vi "Queues fgv.vi"(7 "Modes":T1, 8 "error in (no error)":errorcluster) -> (0 "error in (no error) 2":errorcluster, 1 "DAQ":refnum<queue>, 2 "Camera":refnum<queue>, 3 "Ivium":refnum<queue>)   [LabVIEW 2016]
uses:
  Controls/Queue modes.ctl
  Controls/State control cluster.ctl
  Controls/States.ctl
  Webcam/Controls/Camera queue.ctl
  Webcam/Controls/Camera states.ctl
  DAQ/Controls/DAQ queue.ctl
  DAQ/Controls/Queue states.ctl
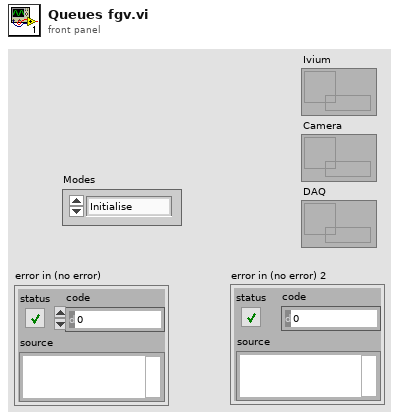
[diagram p1: front panel]
types:
  T1 = typedef "Queue modes.ctl" = enum16{"Initialise", "Destroy", "Get"}
  T2 = typedef "DAQ queue.ctl" = cluster{"Sate":T3, "Data":variant}
  T3 = typedef "Queue states.ctl" = enum16{"Shutdown", "Save data", "Record", "Read", "Setup", "Zero", "Connect", "Initialise"}
  T4 = typedef "Camera queue.ctl" = cluster{"State":T5, "Data":variant}
  T5 = typedef "Camera states.ctl" = enum16{"Initialise", "Setup", "Connect", "Snap", "Close", "Shutdown"}
  T6 = typedef "State control cluster.ctl" = cluster{"State":T7, "Data":variant}
  T7 = typedef "States.ctl" = enum16{"Initialise", "Actuator connection", "Get info", "Send command", "Load method", "Run method", "Save test", "Setup", "Shutdown"}
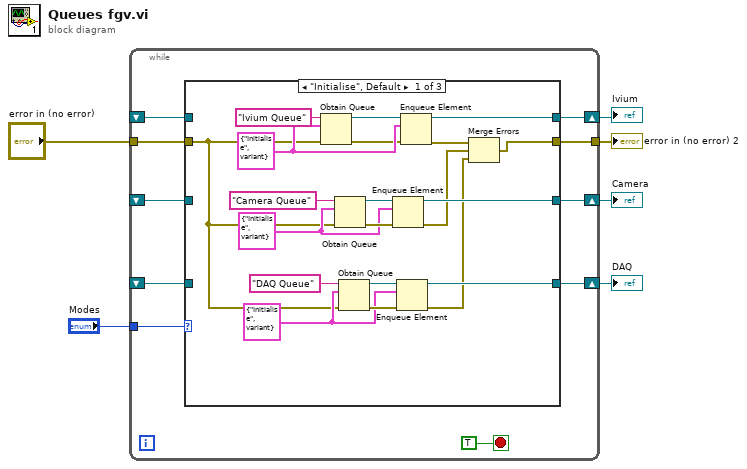
[diagram p0: block diagram]
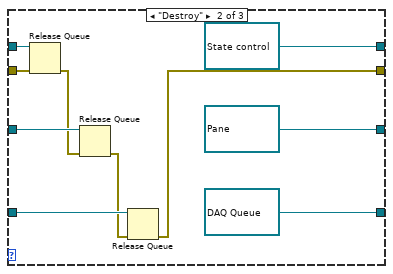
[diagram p2: hidden frame]
diagram:
  n1 = while {
    tunnel: "Modes" -> [w15]
    shift-right: [w14] -> w3
    shift-left: _ -> [w13]
    tunnel: "error in (no error)" -> [w12]
    shift-right: [w11] -> w2
    shift-left: _ -> [w10]
    shift-right: [w9] -> w1
    shift-left: _ -> [w8]
    tunnel: [w7] -> w4
    stop <- TRUE stop-if-true
    n2 = case shown="\"Initialise\", Default" w15 {
      tunnel: [w32 refnum<queue> refnum ("queue out") w50] -> w14
      tunnel: w13 -> [_ w46 w50]
      tunnel: w12 -> [w22 w44 w49]
      tunnel: [w27 refnum<queue> refnum ("queue out") w48] -> w11
      tunnel: w10 -> [_ w43 w48]
      tunnel: [w21 refnum<queue> refnum ("queue out") w47] -> w9
      tunnel: w8 -> [_ w41 w47]
      tunnel: [w17 w39 w49] -> w7
      frame "Initialise", Default {
        w23 = T2 {"Sate"=enum."Initialise", "Data"=variant} ("DAQ Queue")
        w30 = T4 {"State"=enum."Initialise", "Data"=variant}
        w35 = T6 {"State"=enum."Initialise", "Data"=variant} ("State control")
        n3 = Obtain Queue(name (unnamed)="Ivium Queue", element data type=w35, error in (no error)=w22) -> (queue out=w34:refnum<queue>, error out=w33:errorcluster)  [unwired: 2 in, 1 out]
        n4 = Obtain Queue(name (unnamed)="Camera Queue", element data type=w30, error in (no error)=w22) -> (queue out=w28:refnum<queue>, error out=w31:errorcluster)  [unwired: 2 in, 1 out]
        n5 = Obtain Queue(name (unnamed)="DAQ Queue", element data type=w23, error in (no error)=w22) -> (queue out=w26:refnum<queue>, error out=w24:errorcluster)  [unwired: 2 in, 1 out]
        n6 = Enqueue Element(queue=w28, element=w30, error in (no error)=w31) -> (queue out=w27:refnum<queue>, error out=w19:errorcluster)  [unwired: 1 in, 1 out]
        n7 = Enqueue Element(queue=w26, element=w23, error in (no error)=w24) -> (queue out=w21:refnum<queue>, error out=w18:errorcluster)  [unwired: 1 in, 1 out]
        n8 = Enqueue Element(queue=w34, element=w35, error in (no error)=w33) -> (queue out=w32:refnum<queue>, error out=w20:errorcluster)  [unwired: 1 in, 1 out]
        n9 = Merge Errors(w20, w19, w18) -> (w17:errorcluster)
      }
      frame "Destroy" {
        n10 = Release Queue(queue=w46, error in (no error)=w44) -> (error out=w42:errorcluster)  [unwired: 1 in, 2 out]
        n11 = Release Queue(queue=w43, error in (no error)=w42) -> (error out=w40:errorcluster)  [unwired: 1 in, 2 out]
        n12 = Release Queue(queue=w41, error in (no error)=w40) -> (error out=w39:errorcluster)  [unwired: 1 in, 2 out]
      }
      frame "Get" {
      }
    }
  }
  "error in (no error) 2" <- w4
  "Ivium" <- w3
  "Camera" <- w2
  "DAQ" <- w1
